vi "Save Binary format.vi"(5 "action":string="Save", 8 "error in":errorcluster, 10 "file path (use dialog)":path, 11 "data in":sgl[](array[numeric])) -> (0 "error out":errorcluster)   [LabVIEW 2018]
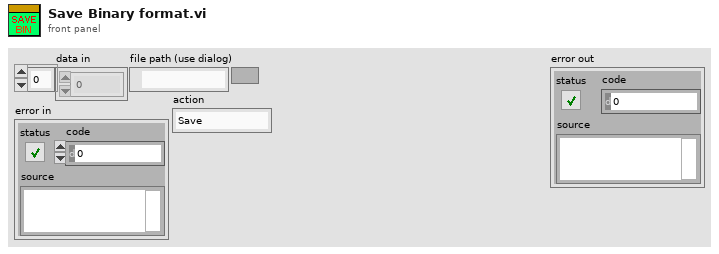
[diagram p1: front panel]
types:
  T1 = enum16{"big-endian, network order", "native, host order", "little-endian"}
  T2 = enum16{"open", "replace", "create", "open or create", "replace or create", "replace or create with confirmation"}
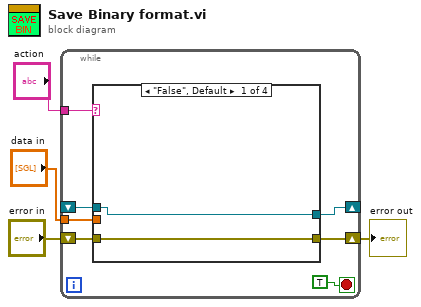
[diagram p0: block diagram]
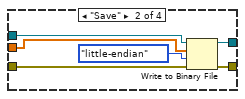
[diagram p2: hidden frame]
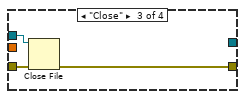
[diagram p3: hidden frame]
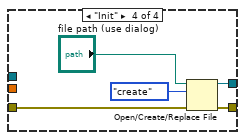
[diagram p4: hidden frame]
diagram:
  n1 = while {
    tunnel: "action" -> [w10]
    tunnel: "data in" -> [w9]
    shift-right: [w7] -> w1
    shift-left: "error in" -> [w8]
    shift-right: [w6] -> _
    shift-left: _ -> [w5]
    stop <- TRUE stop-if-true
    n2 = case shown="\"False\", Default" w10 {
      tunnel: w9 -> [_ w19 _ _]
      tunnel: w8 -> [w13 w18 w22 w25]
      tunnel: [w13 w17 w20 w23] -> w7
      tunnel: [w12 w14 _ w27] -> w6
      tunnel: w5 -> [w12 w15 w21 _]
      frame "False", Default {
      }
      frame "Save" {
        n3 = Write to Binary File(file (use dialog)=w15, data=w19, error in=w18, 9:T1."little-endian" ("byte order (0:big-endian, network order)")) -> (refnum out=w14:refnum<file>, error out=w17:errorcluster)  [unwired: 2 in, 1 out]
      }
      frame "Close" {
        n4 = Close File(refnum=w21, error in=w22) -> (error out=w20:errorcluster)  [unwired: 1 out]
      }
      frame "Init" {
        n5 = Open/Create/Replace File(file path (use dialog)="file path (use dialog)", error in=w25, operation (0:open)=T2."create") -> (refnum out=w27:refnum<file>, error out=w23:errorcluster)  [unwired: 3 in, 1 out]
      }
    }
  }
  "error out" <- w1
